vi "Get Waveform.vi"(8 "error in (no error)":errorcluster, 10 "Tag Path":string, 11 "Logger in.lvclass":refnum<class "Logger.lvclass">) -> (0 "error out":errorcluster, 1 "Buffer Size":i32, 2 "Buffer Waveform":waveform(dbl), 3 "Logger out.lvclass":refnum<class "Logger.lvclass">)   [LabVIEW 2017, in "Logger.lvclass"]
uses:
  Logger.lvclass
  Logger.lvclass/Logger.ctl
  <vilib>/Waveform/WDTOps.llb/WDT Number of Waveform Samples DBL.vi
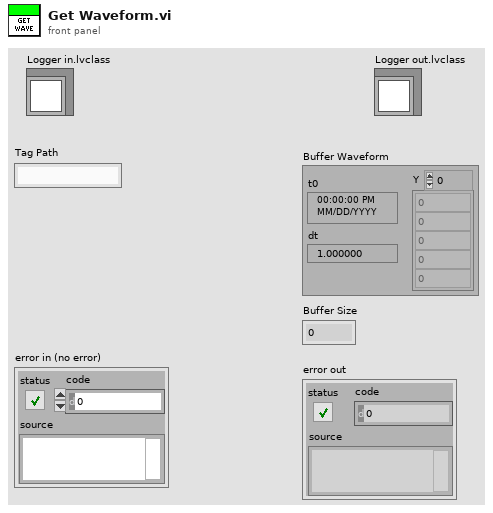
[diagram p1: front panel]
types:
  T1 = cluster{"Tag Reference":refnum<k21>, "Tag Units":string, "Tag Path":string, "Waveform":waveform(dbl), "Log":bool}[]
  T2 = cluster{"Tag Reference":refnum<k21>, "Tag Units":string, "Tag Path":string, "Waveform":waveform(dbl), "Log":bool}
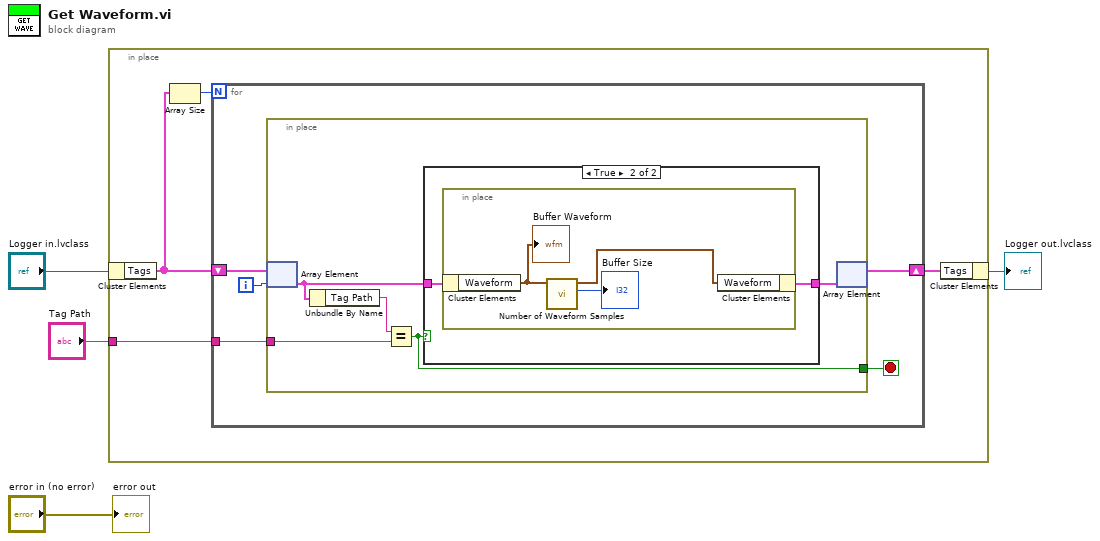
[diagram p0: block diagram]
diagram:
  n1 = in-place {
    in-place-border: "Tag Path" -> [w8]
    n2 = in-place-cluster #1("Logger in.lvclass") -> ("Tags"=w5:T1)
    n3 = Array Size(array=w5) -> (size(s)=w6:i32)
    n4 = for {
      N: w6 -> [_]
      tunnel: w8 -> [w13]
      shift-right: [w10] -> w7
      shift-left: w5 -> [w12]
      i -> [w11]
      stop <- w9 stop-if-true
      n5 = in-place {
        in-place-border: w13 -> [w15]
        in-place-border: [w14] -> w9
        n6 = in-place-array #2(w12, w11) -> (w17:T2)
        n7 = Unbundle By Name(w17) -> ("Tag Path"=w16:string)
        n8 = Equal?(x=w16, y=w15) -> (x = y?=w14:bool)
        n9 = case shown="True" w14 {
          tunnel: w17 -> [w19 w21]
          tunnel: [w19 w20] -> w18
          frame False {
          }
          frame True {
            n10 = in-place {
              n11 = in-place-cluster #3(w21) -> ("Waveform"=w24:waveform(dbl))
              "Buffer Waveform" <- w24
              n12 = call-poly <vilib>:"Number of Waveform Samples.vi"("waveform in"=w24) -> ("number of samples"=→"Buffer Size":i32, "waveform out"=w23:waveform(dbl))  [unwired: 8 in, 1 out]
              n13 = in-place-cluster #3("Waveform"=w23) -> (w20:T2)
            }
          }
        }
        n14 = in-place-array #2(w18) -> (w10:T1)  [unwired: 1 out]
      }
    }
    n15 = in-place-cluster #1("Tags"=w7) -> (→"Logger out.lvclass":refnum<class "Logger.lvclass">)
  }
  "error out" <- "error in (no error)"
